vi "Close.vi"(8 "error in (no error)":errorcluster caption="错误输入（无错误）", 11 "DevControl 输入":refnum<class "DevControl.lvclass"> caption="DNL_LabVIEW Object in") -> (0 "error out":errorcluster caption="错误输出", 3 "DevControl 输出":refnum<class "DevControl.lvclass"> caption="DNL_LabVIEW Object out")   [LabVIEW 2012, in "DevControl.lvclass"]
uses:
  DevControl.lvclass
  DevControl.lvclass/DevControl.ctl
  Libs/Serial/Serial.lvclass
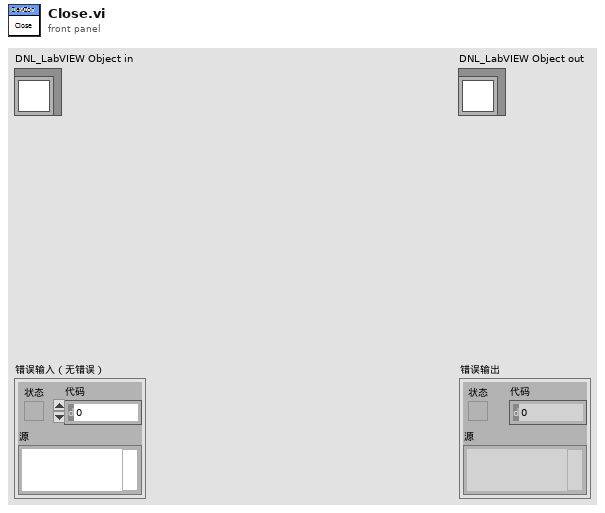
[diagram p1: front panel]
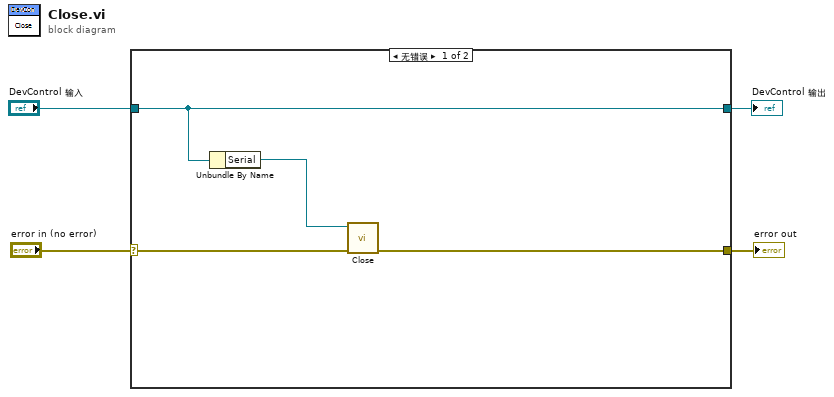
[diagram p0: block diagram]
diagram:
  n1 = case shown="无错误" "error in (no error)" {
    selector: "error in (no error)" -> [w8 w10]
    tunnel: [w6 w10] -> w3
    tunnel: [w5 w9] -> w1
    tunnel: "DevControl 输入" -> [w5 w9]
    frame No Error {
      n2 = Unbundle By Name(w5) -> ("Serial"=w7:refnum<class "Serial.lvclass">)
      n3 = call-dynamic "Close.vi"("error in (no error)"=w8, "Serial 输入"=w7) -> ("error out"=w6:errorcluster)  [unwired: 8 in, 1 out]
    }
    frame Error {
    }
  }
  "error out" <- w3
  "DevControl 输出" <- w1
